vi "File Format Converter.vi"(8 "Error In":errorcluster, 10 "Configuration":T1={"New start time"=nan, "New end time"=nan, "Output file format"=enum."ASCII", "Save ASCII column names"=TRUE, "Prepend binary array size"=FALSE, "buffer size (-1: all)"=100000, "Channels"=[], "Group"="p", "New dt"=nan} {"buffer size (-1: all)" format="%.0p"; "New start time" format="%#_10p"}, 11 "File":path) -> (0 "Error Out":errorcluster, 2 "New file out":path, 3 "File out":path)   [LabVIEW 2021]
uses:
  Format Converter Configuration.ctl
  <vilib>/Utility/file.llb/Write Delimited Spreadsheet (DBL).vi
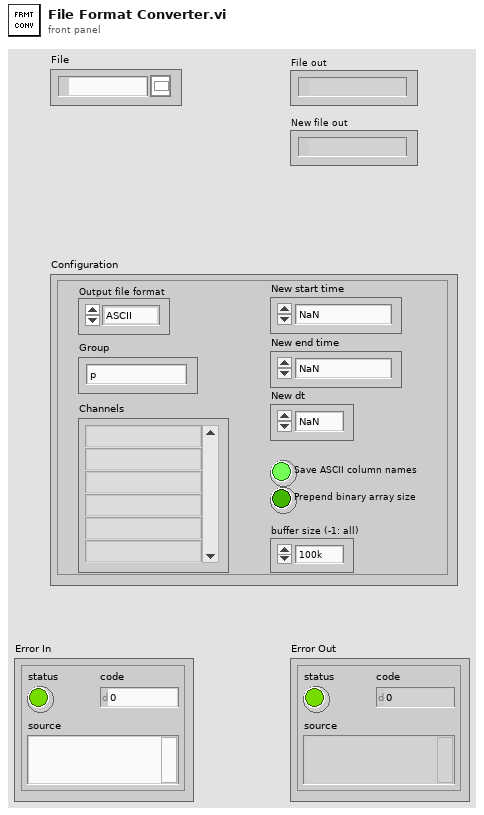
[diagram p1: front panel]
types:
  T1 = typedef "Format Converter Configuration.ctl" = cluster{"New start time":dbl, "New end time":dbl, "Output file format":enum16{"HDF5", "ASCII", "BINARY", "TDMS"}, "Save ASCII column names":bool, "Prepend binary array size":bool, "buffer size (-1: all)":i64, "Channels":string[], "Group":string, "New dt":dbl}
  T2 = enum16{"open", "open or create", "create or replace", "create", "open (read-only)"}
  T3 = enum16{"open", "replace", "create", "open or create", "replace or create", "replace or create with confirmation"}
  T4 = typedef "TDMS channel info.ctl" = cluster{"t0":timestamp, "dt":dbl, "Channel length":i64}
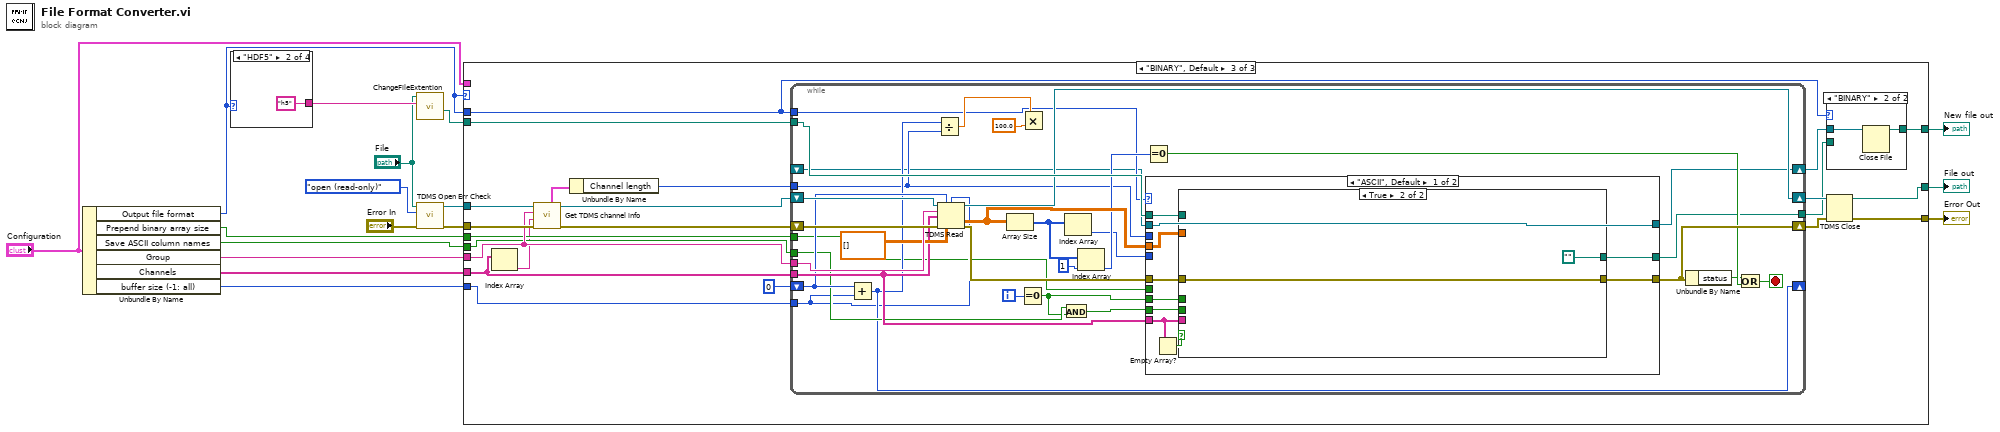
[diagram p0: block diagram]
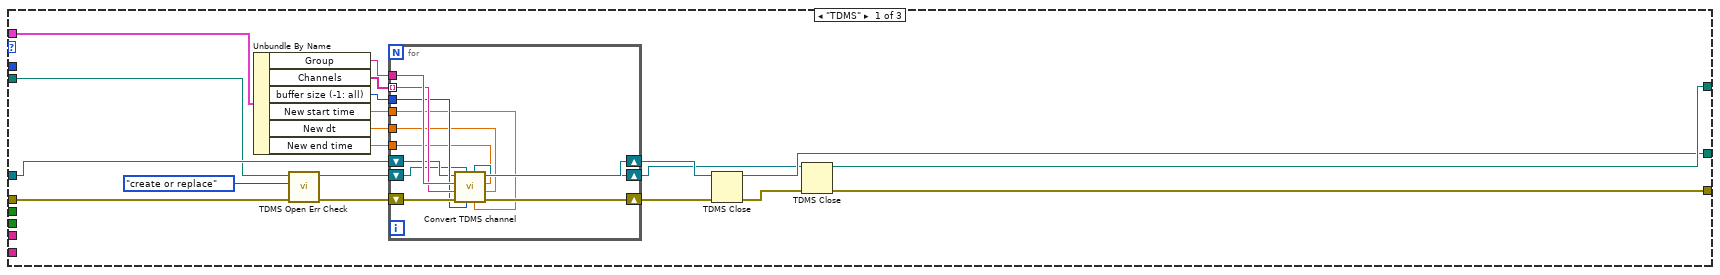
[diagram p2: hidden frame]
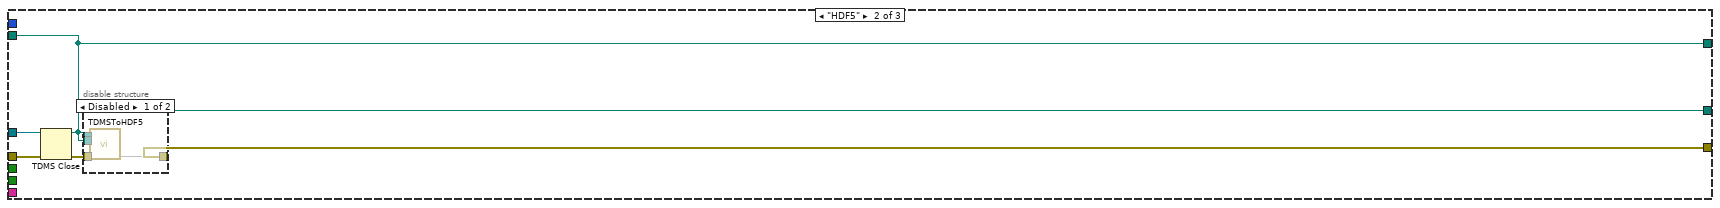
[diagram p3: hidden frame]
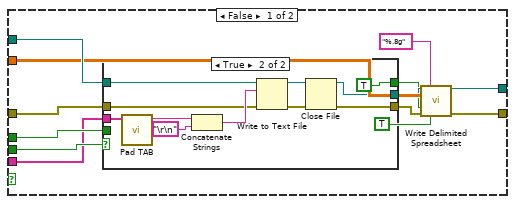
[diagram p6: hidden frame]
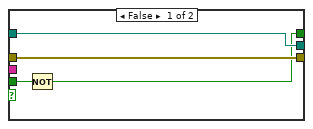
[diagram p7: hidden frame]
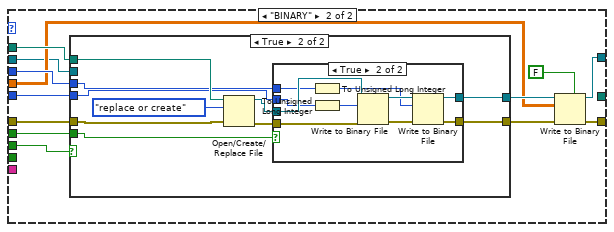
[diagram p8: hidden frame]
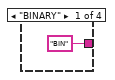
[diagram p11: hidden frame]
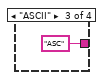
[diagram p12: hidden frame]
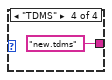
[diagram p13: hidden frame]
diagram:
  n1 = Unbundle By Name("Configuration") -> ("Output file format"=w8:enum16{"HDF5", "ASCII", "BINARY", "TDMS"}, "Prepend binary array size"=w10:bool, "Save ASCII column names"=w11:bool, "Group"=w13:string, "Channels"=w14:string[], "buffer size (-1: all)"=w12:i64)
  n2 = case shown="\"HDF5\"" w8 {
    tunnel: ["BIN" ("New Extention") "h5" ("New Extention") "ASC" ("New Extention") "new.tdms" ("New Extention")] -> w17
    frame "BINARY" {
    }
    frame "HDF5" {
    }
    frame "ASCII" {
    }
    frame "TDMS" {
    }
  }
  n3 = call "ChangeFileExtention.vi"("New extension"=w17, "File Path"="File") -> ("Path with new extension"=w16:path)  [unwired: 4 in, 5 out]
  n4 = call "TDMS Open Err Check.vi"("Error In"="Error In", "operation (0:open)"=T2."open (read-only)", "File Path Control"="File") -> ("Error Out"=w1:errorcluster, "tdms file out"=w2:refnum<k34>)  [unwired: 6 in, 1 out]
  n5 = case shown="\"BINARY\", Default" w8 {
    tunnel: w1 -> [w25 w58 w86]
    tunnel: w2 -> [w41 w59 w85]
    tunnel: w16 -> [w27 w54 w84]
    tunnel: [w37 w56 w83] -> w15
    tunnel: w8 -> [_ _ w82]
    tunnel: w13 -> [_ _ w81]
    tunnel: w14 -> [_ _ w80]
    tunnel: w12 -> [_ _ w79]
    tunnel: w11 -> [_ _ w78]
    tunnel: w10 -> [_ _ w77]
    tunnel: "Configuration" -> [w33 _ _]
    tunnel: [w29 w54 w67] -> w7
    tunnel: [w28 w55 w65] -> w6
    frame "TDMS" {
      n6 = Unbundle By Name(w33) -> ("Group"=w36:string, "Channels"=w35:string[], "buffer size (-1: all)"=w34:i64, "New start time"=w32:dbl, "New dt"=w31:dbl, "New end time"=w30:dbl)
      n7 = call "TDMS Open Err Check.vi"("Error In"=w25, "operation (0:open)"=T2."create or replace", "File Path Control"=w27) -> ("Error Out"=w24:errorcluster, "tdms file out"=w23:refnum<k34>)  [unwired: 6 in, 1 out]
      n8 = for {
        shift-right: [w45] -> w40
        shift-left: w24 -> [w51]
        shift-right: [w48] -> w39
        shift-left: w41 -> [w49]
        shift-right: [w46] -> w22
        shift-left: w23 -> [w47]
        tunnel: w34 -> [w50]
        tunnel: w36 -> [w53]
        tunnel: w35 -> [w52] mode=indexing
        tunnel: w32 -> [w44]
        tunnel: w31 -> [w43]
        tunnel: w30 -> [w42]
        n9 = call "Convert TDMS channel.vi"("dt"=w43, "End time"=w42, "Start time"=w44, "buffer size (-1: all)"=w50, "Output tdms ref"=w47, "Error In"=w51, "Channel name"=w52, "Group name"=w53, "Input tdms ref"=w49) -> ("Error Out"=w45:errorcluster, "Input tdms ref out"=w48:refnum<k34>, "Output tdms ref out"=w46:refnum<k34>)
      }
      n10 = TDMS Close(8:w40, 11:w39) -> (0:w38:errorcluster, 3:w28:path)
      n11 = TDMS Close(8:w38, 11:w22) -> (0:w37:errorcluster, 3:w29:path)
    }
    frame "HDF5" {
      n12 = TDMS Close(8:w58, 11:w59) -> (0:w57:errorcluster, 3:w55:path)
      n13 = disable-structure shown="Disabled" {
        disable-tunnel: w57 -> [w63 w64]
        disable-tunnel: [w62 w64] -> w56
        disable-tunnel: w55 -> [w61 _]
        disable-tunnel: w54 -> [w60 _]
        frame Disabled {
          n14 = call "TDMSToHDF5.vi"(8:w63, 10:w60, 11:w61) -> (0:w62)  [unwired: 8 in]
        }
        frame Enabled {
        }
      }
    }
    frame "BINARY", Default {
      n15 = Index Array(array=w80) -> (element=w72:string)  [unwired: 1 in]
      n16 = call "Get TDMS channel info.vi"("error in"=w86, "Channel name"=w72, "group name"=w81, "tdms file"=w85) -> ("error out"=w68:errorcluster, "tdms file out"=w71:refnum<k34>, "TDMS channel info"=w70:T4)  [unwired: 3 in, 2 out]
      n17 = Unbundle By Name(w70) -> ("Channel length"=w69:i64)
      n18 = while {
        tunnel: w81 -> [w120]
        tunnel: w80 -> [w117]
        tunnel: w78 -> [w110]
        tunnel: w84 -> [w116]
        shift-right: [w99] -> _
        shift-left: i64 0 -> [w113]
        shift-right: [w108] -> w74
        shift-left: w71 -> [w118]
        shift-right: [w105] -> w75
        shift-left: w68 -> [w121]
        tunnel: w69 -> [w95]
        tunnel: w82 -> [w98]
        shift-right: [w94] -> w73
        shift-left: _ -> [w93]
        tunnel: w79 -> [w92]
        tunnel: w77 -> [w91]
        tunnel: [w90] -> w66
        i -> [w112]
        stop <- w104 stop-if-true
        n19 = Add(x=w113, y=w92) -> (x+y=w99:i64)
        n20 = Divide(x=w99, y=w95) -> (x/y=w101:dbl)
        n21 = TDMS Read(0:w118, 1:w113, 2:w92, 5:w120, 7:w117, 11:w121, 12:dbl[][] []) -> (4:w108:refnum<k34>, 10:w115:dbl[][], 15:w107:errorcluster)  [unwired: 1 in, 3 out]
        n22 = Array Size(array=w115) -> (size(s)=w97:i32[])
        n23 = Equal To 0?(x=w112) -> (x = 0?=w109:bool)
        n24 = Multiply(x=w101, y=100.0) -> ()  [unwired: 1 out]
        n25 = And(x=w110, y=w109) -> (x .and. y?=w111:bool)
        n26 = Index Array(array=w97) -> (element=w96:i32)  [unwired: 1 in]
        n27 = Index Array(array=w97, index=1) -> (element=w114:i32)
        n28 = Equal To 0?(x=w114) -> (x = 0?=w103:bool)
        n29 = case shown="\"ASCII\", Default" w98 {
          tunnel: w117 -> [w131 _]
          tunnel: w116 -> [w130 w173]
          tunnel: w115 -> [w125 w167]
          tunnel: w111 -> [w129 _]
          tunnel: w109 -> [w128 w174]
          tunnel: w107 -> [w127 w172]
          tunnel: [w124 w166] -> w105
          tunnel: w96 -> [_ w171]
          tunnel: w95 -> [_ w170]
          tunnel: [w126 w165] -> w94
          tunnel: w93 -> [w126 w164]
          tunnel: w91 -> [_ w162]
          tunnel: [w123 _] -> w90
          frame "ASCII", Default {
            n30 = Empty Array?(array=w131) -> (empty?=w122:bool)
            n31 = case shown="True" w122 {
              tunnel: w131 -> [w132 _]
              tunnel: w130 -> [w144 _]
              tunnel: w129 -> [w143 _]
              tunnel: w128 -> [w142 _]
              tunnel: w127 -> [w141 w161]
              tunnel: w125 -> [w140 _]
              tunnel: [w135 w161] -> w124
              tunnel: [w133 path ""] -> w123
              frame False {
                n32 = case shown="True" w143 {
                  tunnel: [w145 TRUE] -> w136
                  tunnel: [w147 w153] -> w134
                  tunnel: w132 -> [_ w157]
                  tunnel: [w148 w151] -> w137
                  tunnel: w141 -> [w147 w150]
                  tunnel: w144 -> [w148 w149]
                  tunnel: w142 -> [w146 _]
                  frame False {
                    n33 = Not(x=w146) -> (.not. x?=w145:bool)
                  }
                  frame True {
                    n34 = call "Pad TAB.vi"("Input String Array"=w157) -> ("Output String"=w158:string)  [unwired: 10 in]
                    n35 = Concatenate Strings(w158, "\r\n") -> (w156:string)
                    n36 = Write to Text File(file (use dialog)=w149, text=w156, error in=w150) -> (refnum out=w152:refnum<file>, error out=w154:errorcluster)  [unwired: 2 out]
                    n37 = Close File(refnum=w152, error in=w154) -> (path=w151:path, error out=w153:errorcluster)
                  }
                }
                n38 = call-poly <vilib>:"Write Delimited Spreadsheet.vi"("file path (dialog if empty)"=w137, "format (%.3f)"="%.8g", "2D data"=w140, "append to file? (new file:F)"=w136, "error in (no error)"=w134, "transpose? (no:F)"=TRUE) -> ("new file path (Not A Path if cancelled)"=w133:path, "error out"=w135:errorcluster)  [unwired: 8 in]
              }
              frame True {
              }
            }
          }
          frame "BINARY" {
            n39 = case shown="True" w174 {
              tunnel: w173 -> [_ w186]
              tunnel: w172 -> [w175 w185]
              tunnel: w171 -> [_ w181]
              tunnel: w170 -> [_ w180]
              tunnel: [w175 w179] -> w169
              tunnel: [w176 w178] -> w168
              tunnel: w164 -> [w176 _]
              tunnel: w162 -> [_ w177]
              frame False {
              }
              frame True {
                n40 = Open/Create/Replace File(file path (use dialog)=w186, error in=w185, operation (0:open)=T3."replace or create") -> (refnum out=w182:refnum<file>, error out=w183:errorcluster)  [unwired: 3 in, 1 out]
                n41 = case shown="True" w177 {
                  tunnel: w183 -> [w188 w198]
                  tunnel: w182 -> [w187 w197]
                  tunnel: w181 -> [_ w196]
                  tunnel: w180 -> [_ w193]
                  tunnel: [w188 w192] -> w179
                  tunnel: [w187 w191] -> w178
                  frame False {
                  }
                  frame True {
                    n42 = To Unsigned Long Integer(number=w193) -> (unsigned 32bit integer=w189:u32)
                    n43 = To Unsigned Long Integer(number=w196) -> (unsigned 32bit integer=w190:u32)
                    n44 = Write to Binary File(file (use dialog)=w197, data=w190, error in=w198) -> (refnum out=w194:refnum<file>, error out=w195:errorcluster)  [unwired: 3 in, 1 out]
                    n45 = Write to Binary File(file (use dialog)=w194, data=w189, error in=w195) -> (refnum out=w191:refnum<file>, error out=w192:errorcluster)  [unwired: 3 in, 1 out]
                  }
                }
              }
            }
            n46 = Write to Binary File(file (use dialog)=w168, data=w167, error in=w169, 5:FALSE ("prepend array or string size? (T)")) -> (refnum out=w165:refnum<file>, error out=w166:errorcluster)  [unwired: 2 in, 1 out]
          }
        }
        n47 = Unbundle By Name(w105) -> ("status"=w102:bool)
        n48 = Or(x=w102, y=w103) -> (x .or. y?=w104:bool)
      }
      n49 = case shown="\"BINARY\"" w82 {
        tunnel: w73 -> [_ w89]
        tunnel: [w87 w88] -> w67
        tunnel: w66 -> [w87 _]
        frame "ASCII", Default {
        }
        frame "BINARY" {
          n50 = Close File(refnum=w89) -> (path=w88:path)  [unwired: 1 in, 1 out]
        }
      }
      n51 = TDMS Close(8:w75, 11:w74) -> (0:w83:errorcluster, 3:w65:path)
    }
  }
  "Error Out" <- w15
  "File out" <- w6
  "New file out" <- w7
